vi "SINAD Analyzer N Chan.vi"(6 "advanced search":T4={"approx freq. (optional)"=-1.0, "search (+/- % of Fsampl.)"=5.0} {"search (+/- % of Fsampl.)" format="%0.2p"; "approx freq. (optional)" format="%0.2p"}, 8 "error in (no error)":errorcluster, 10 "export  mode":T2(ring), 11 "signals in":waveform(dbl)[](array[waveform])) -> (0 "error out":errorcluster, 1 "THD Plus Noise":dbl[](array[numeric]) format="%.2p", 2 "SINAD (dB)":dbl[](array[numeric]) format="%.2p", 3 "detected fundamental \nfrequencies":dbl[](array[numeric]) format="%.2p", 4 "measurements info":T3(array[cluster]) {"uncertainty" format="%0.2p"}, 5 "exported signals":T1(array[cluster]) {"exported spectrum (dB)"."dB Spectrum (Hann)" format="%.2p"; "exported spectrum (dB)"."df" format="%.2p"; "exported spectrum (dB)"."f0" format="%.2p"})   [LabVIEW 2020, in "NI_MAPro.lvlib"]
doc: "Takes a signal in and performs a full Signal in Noise and Distortion (SINAD) analysis, including measuring the fundamental frequency tone and returning the fundamental frequency and SINAD level in dB. Wire data to the <B>signal in</B> input to determine the polymorphic instance to use or manually select the instance."
uses:
  NI_MAPro.lvlib
  NI_MABase.lvlib
panel:
  # "Signal / Noise & Distortion (SINAD) Analyzer"
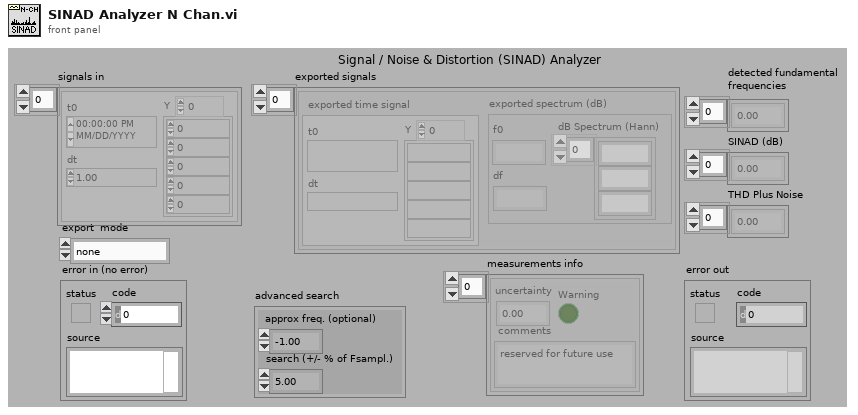
[diagram p1: front panel]
types:
  T1 = cluster{"exported time signal":waveform(dbl), "exported spectrum (dB)":cluster{"f0":dbl, "df":dbl, "dB Spectrum (Hann)":dbl[]}}[]
  T2 = enum16{"none", "input signal", "fundamental signal", "residual signal"}
  T3 = cluster{"uncertainty":dbl, "Warning":bool, "comments":string}[]
  T4 = cluster{"approx freq. (optional)":dbl, "search (+/- % of Fsampl.)":dbl}
  T5 = cluster{"uncertainty":dbl, "Warning":bool, "comments":string}
  T6 = cluster{"exported time signal":waveform(dbl), "exported spectrum (dB)":cluster{"f0":dbl, "df":dbl, "dB Spectrum (Hann)":dbl[]}}
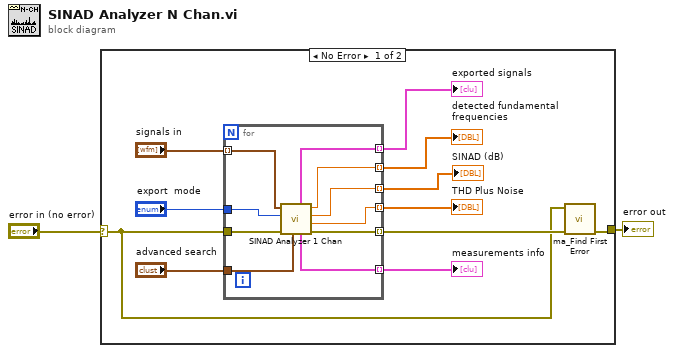
[diagram p0: block diagram]
diagram:
  n1 = case shown="No Error" "error in (no error)" {
    selector: "error in (no error)" -> [w6 w24]
    tunnel: [w7 w24] -> w2
    frame No Error {
      n2 = for {
        tunnel: [w18] -> w13 mode=indexing
        tunnel: [w23] -> w12 mode=indexing
        tunnel: [w20] -> w11 mode=indexing
        tunnel: "signals in" -> [w17] mode=indexing
        tunnel: [w19] -> w9 mode=indexing
        tunnel: w6 -> [w16]
        tunnel: [w22] -> w8 mode=indexing
        tunnel: [w21] -> w5 mode=indexing
        tunnel: "export  mode" -> [w15]
        tunnel: "advanced search" -> [w14]
        n3 = call "SINAD Analyzer 1 Chan.vi"("advanced search"=w14, "error in (no error)"=w16, "export  mode"=w15, "signal in"=w17) -> ("error out"=w22:errorcluster, "THD Plus Noise"=w21:dbl, "SINAD (dB)"=w20:dbl, "detected fundamental\nfrequency"=w19:dbl, "measurement info"=w23:T5, "exported signals"=w18:T6)  [unwired: 2 out]
      }
      "detected fundamental \nfrequencies" <- w9
      "SINAD (dB)" <- w11
      "measurements info" <- w12
      "exported signals" <- w13
      "THD Plus Noise" <- w5
      n4 = call "ma_Find First Error.vi"("error array in"=w8, "error in 1 (no error)"=w6) -> ("error out"=w7:errorcluster)  [unwired: 2 in, 3 out]
    }
    frame Error {
    }
  }
  "error out" <- w2
